vi "DS345_BurstMode.contents.vi"() -> ()   [LabVIEW 2014, in "DS345_BurstMode.lvlib"]
doc: "Contains the top level VIs of this class. Needed for debugging and building applications."
uses:
  DS345_BurstMode.lvlib
panel:
  out "error out":errorcluster
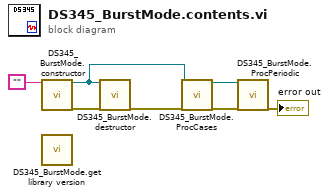
[diagram p0: block diagram]
diagram:
  n1 = call "DS345_BurstMode.constructor.vi"("name"="") -> ("i ref out"=w5:refnum<vi>, "error out"=w4:errorcluster)  [unwired: 16 in, 1 out]
  n2 = call "DS345_BurstMode.get library version.vi"() -> ()  [unwired: 1 in, 1 out]
  n3 = call "DS345_BurstMode.destructor.vi"("i ref in"=w5, "error in (no error)"=w4) -> ("error out"=w3:errorcluster)  [unwired: 17 in]
  n4 = call "DS345_BurstMode.ProcCases.vi"("i ref in"=w5, "error in (no error)"=w3) -> ("i ref out"=w7:refnum<vi>, "error out"=w2:errorcluster)  [unwired: 15 in, 1 out]
  n5 = call "DS345_BurstMode.ProcPeriodic.vi"("i ref in"=w7, "error in (no error)"=w2) -> ("error out"=→"error out":errorcluster)  [unwired: 15 in, 2 out]
